vi "CAENHV Test Bd Presence.vi"(8 "error in (no error)":errorcluster, 10 "slot":u16, 11 "handle":i32) -> (0 "error out":errorcluster, 2 "SerNum":u16, 3 "NrofCh":u16, 5 "Description":string, 7 "Model":string)   [LabVIEW 2009, in "CAENHVWrapper.lvlib"]
doc: "CAENHVLIB_API CAENHVRESULT CAENHV_TestBdPresence(int handle, \n ushort slot, ushort *NrofCh, char **Model, char **Description, ushort *SerNum, \n uchar *FmwRelMin, uchar *FmwRelMax);"
uses:
  <userlib>/CAENHVWrapper/CAENHVWrapper.lvlib
  <vilib>/Utility/importsl/GetValueByPointer/GetValueByPointer.xnode
  <vilib>/Utility/importsl/GetValueByPointer/datatype.ctl
  <userlib>/CAENHVWrapper/CAENHVWrapper.dll
  resource/lvimptsl.dll
panel:
  out "FmwRelMax":string
  out "FmwRelMin":string
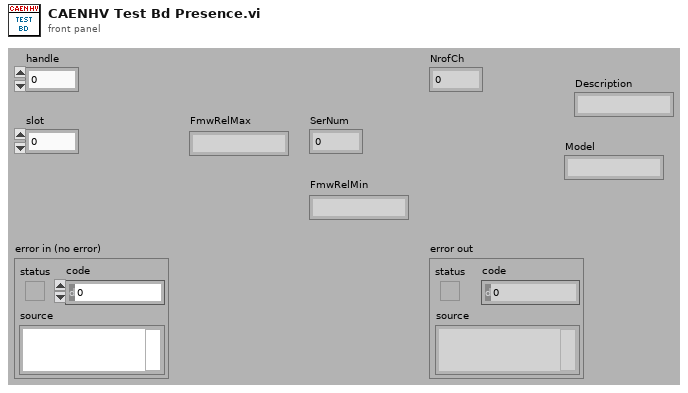
[diagram p1: front panel]
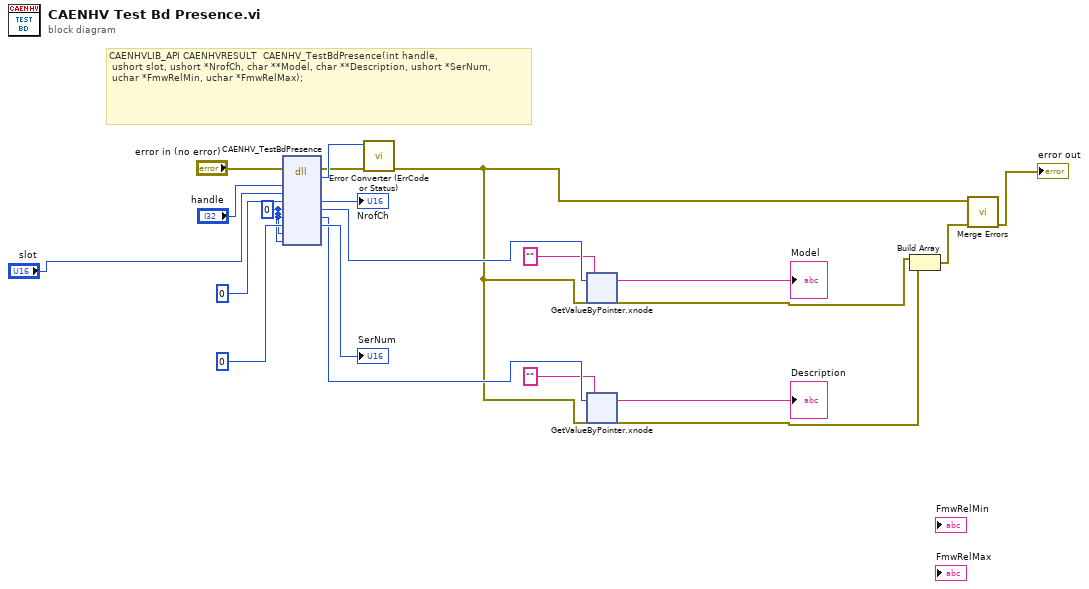
[diagram p0: block diagram]
diagram:
  w14 = i64 0 ("Model")
  # "CAENHVLIB_API CAENHVRESULT  CAENHV_TestBdPresence(int handle, \n ushort slot, ushort *NrofCh, char **Model, char **Description, ushort *SerNum, \n uchar *FmwRelMin, uchar *FmwRelMax);"
  n1 = dll-call lib="C:/Program Files/National Instruments/LabVIEW 2009/user.lib/CAENHVWrapper/CAENHVWrapper.*" fn="CAENHV_TestBdPresence"(error in="error in (no error)", "handle"="handle", "slot"="slot", "NrofCh"=u16 0, "Model"=w14, "Description"=w14, "SerNum"=u16 0, "FmwRelMin"=w14, "FmwRelMax"=w14) -> (error out=w15:errorcluster, "return type"=w16:i32, "NrofCh"=→"NrofCh":u16, "Model"=w13:i64, "Description"=w11:i64, "SerNum"=→"SerNum":u16)  [unwired: 6 in, 1 out]
  n2 = call <userlib>:"Error Converter (ErrCode or Status).vi"("error in (no error)"=w15, "error code"=w16) -> ("error out"=w5:errorcluster)  [unwired: 9 in]
  n3 = xnode "GetValueByPointer.xnode"("Pointer"=w13, "InputType"="", "ErrorIn"=w5) -> ("Output"=→"Model":string, "ErrorOut"=w8:errorcluster)  [unwired: 1 in]
  n4 = xnode "GetValueByPointer.xnode"("Pointer"=w11, "InputType"="", "ErrorIn"=w5) -> ("Output"=→"Description":string, "ErrorOut"=w7:errorcluster)  [unwired: 1 in]
  n5 = Build Array(w8, w7) -> (w6:errorcluster[])
  n6 = call <vilib>:"Merge Errors.vi"("error array in"=w6, "error in 1 (no error)"=w5) -> ("error out"=→"error out":errorcluster)  [unwired: 5 in]
